vi "ReadTextUntilError.vi"(8 "error in (no error)":errorcluster, 11 "Byte Stream File in":refnum<file>) -> (0 "error out":errorcluster, 1 "refnum out":refnum<file>, 3 "Array":dbl[](array[numeric]))   [LabVIEW 2013]
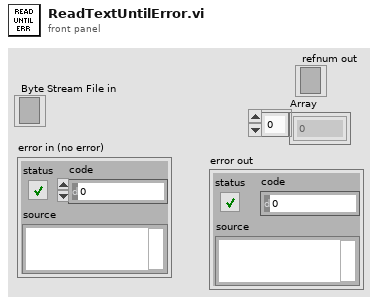
[diagram p1: front panel]
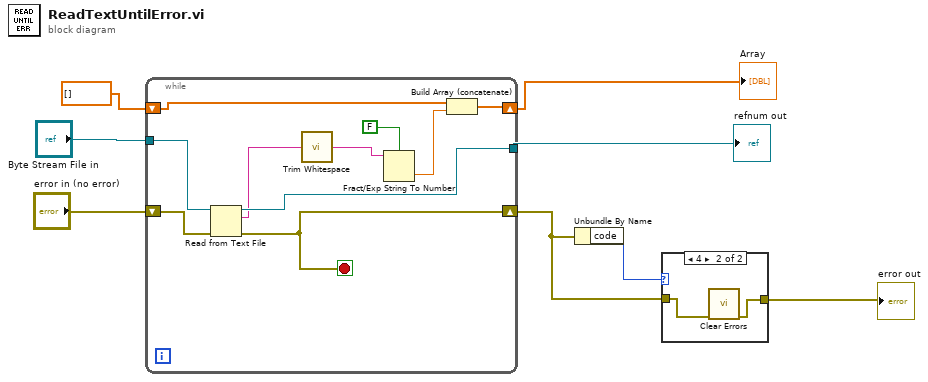
[diagram p0: block diagram]
diagram:
  n1 = while {
    tunnel: "Byte Stream File in" -> [w18]
    shift-right: [w17] -> w1
    shift-left: dbl[] [] -> [w11]
    tunnel: [w16] -> w7
    shift-right: [w14] -> w3
    shift-left: "error in (no error)" -> [w15]
    stop <- w14 stop-if-true
    n2 = Read from Text File(file (use dialog)=w18, error in=w15) -> (refnum out=w16:refnum<file>, text=w13:string, error out=w14:errorcluster)  [unwired: 2 in, 1 out]
    n3 = call <vilib>:"Trim Whitespace.vi"("string"=w13) -> ("trimmed string"=w10:string)  [unwired: 1 in]
    n4 = Fract/Exp String To Number(use system decimal point (T)=FALSE, string=w10) -> (number=w12:dbl)  [unwired: 2 in, 1 out]
    n5 = Build Array (concatenate)(w11, w12) -> (w17:dbl[])
  }
  "refnum out" <- w7
  "Array" <- w1
  n6 = Unbundle By Name(w3) -> ("code"=w5:i32)
  n7 = case shown="4" w5 {
    tunnel: w3 -> [w19 w21]
    tunnel: [w19 w20] -> w4
    frame 1, Default {
    }
    frame 4 {
      n8 = call <vilib>:"Clear Errors.vi"("error in (no error)"=w21) -> ("error out"=w20:errorcluster)  [unwired: 6 in]
    }
  }
  "error out" <- w4
